vi "AnaBuse_Q1.vi"() -> ()   [LabVIEW 2019]
uses:
  <vilib>/measure/matone.llb/Extract Multiple Tone Information 1 Chan.vi
  <vilib>/measure/NI_MAPro.lvlib
panel:
  out "DHT máximo de  de 10%":bool
  out "DHT":dbl
  in  "stop":bool
  in  "LIGAR":bool
  in  "file path":path=path "C:/lista2.tdms"
  out "SINAL DE TENSAO DA REDE":waveform(dbl)(graph)
  out "multiple tone information":T1(array[cluster]) {"detected phase (deg)" format="%_6g"; "detected amplitude" format="%_6p"; "detected frequency" format="%_6p"}
  # "DHT está dentro das normas?"
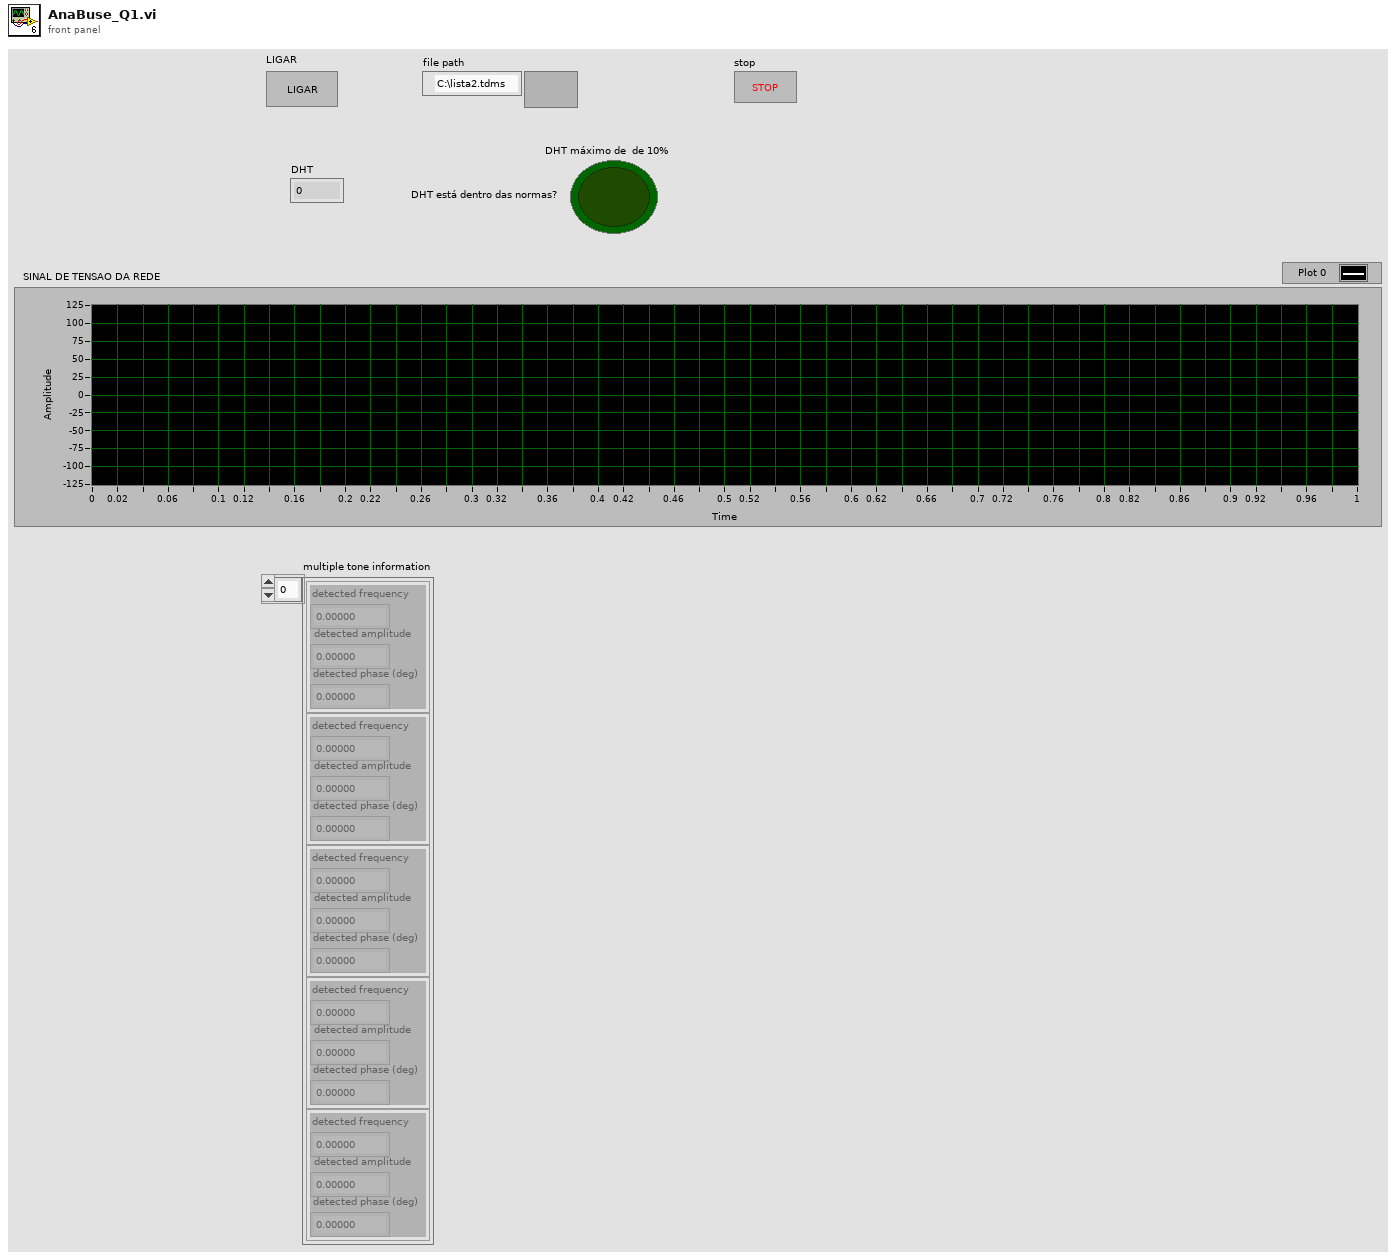
[diagram p1: front panel]
types:
  T1 = cluster{"detected frequency":dbl, "detected amplitude":dbl, "detected phase (deg)":dbl}[]
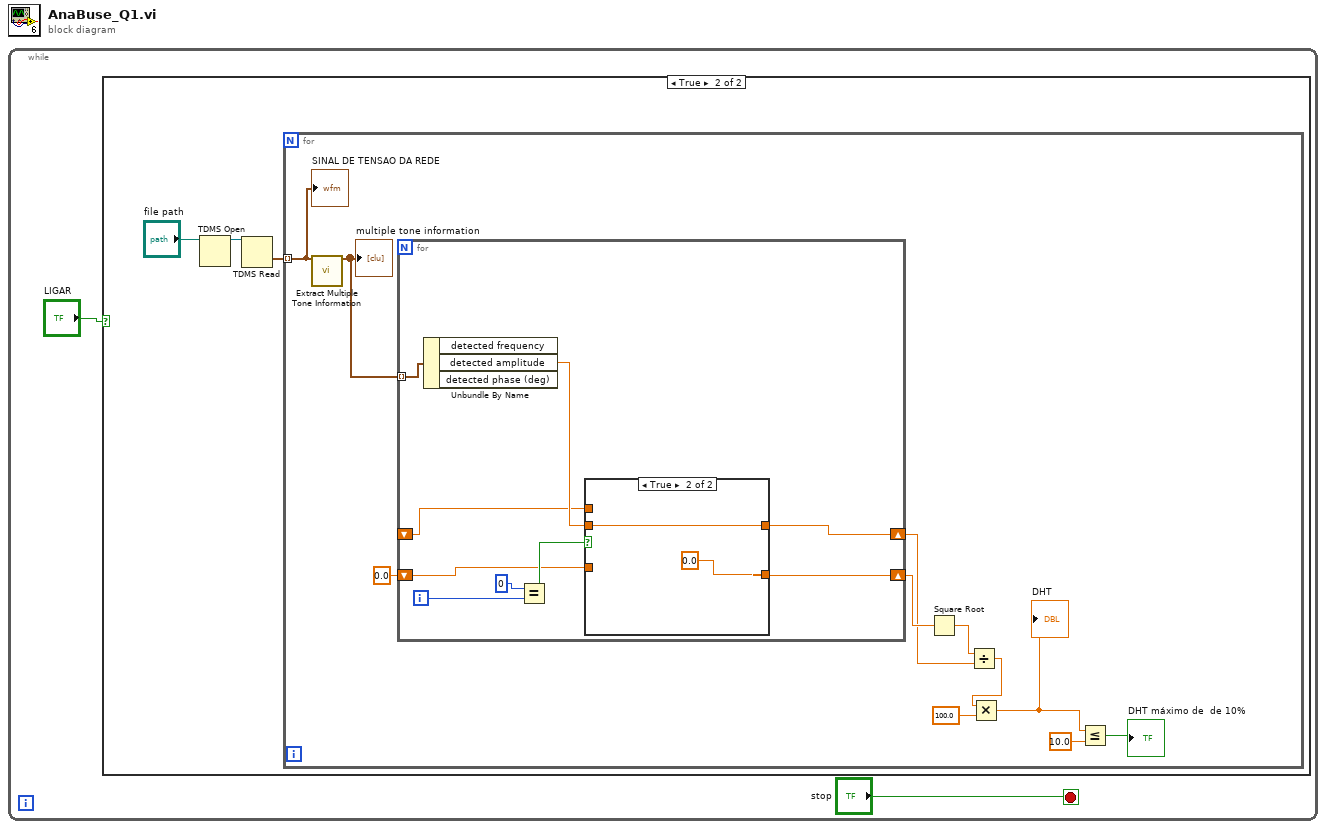
[diagram p0: block diagram]
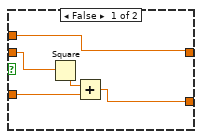
[diagram p3: hidden frame]
diagram:
  n1 = while {
    stop <- "stop" stop-if-true
    n2 = case shown="True" "LIGAR" {
      frame False {
      }
      frame True {
        n3 = TDMS Open(11:"file path") -> (3:w4:refnum<k34>)  [unwired: 6 in, 1 out]
        n4 = TDMS Read(0:w4) -> (10:w3:waveform(dbl)[])  [unwired: 7 in, 5 out]
        n5 = for {
          tunnel: w3 -> [w16] mode=indexing
          n6 = call-poly <vilib>:"Extract Multiple Tone Information.vi"("time signal in"=w16) -> ("multiple tone information"=w15:T1)  [unwired: 12 in, 2 out]
          "multiple tone information" <- w15
          n7 = for {
            tunnel: w15 -> [w25] mode=indexing
            shift-right: [w20] -> w14
            shift-left: 0.0 -> [w19]
            shift-right: [w18] -> w11
            shift-left: _ -> [w17]
            i -> [w22]
            n8 = Unbundle By Name(w25) -> ("detected amplitude"=w24:dbl)  [unwired: 2 out]
            n9 = Equal?(x=0, y=w22) -> (x = y?=w23:bool)
            n10 = case shown="True" w23 {
              tunnel: w24 -> [w30 w32]
              tunnel: [w29 0.0] -> w20
              tunnel: w19 -> [w27 _]
              tunnel: [w26 w32] -> w18
              tunnel: w17 -> [w26 _]
              frame False {
                n11 = Square(x=w30) -> (x^2=w28:dbl)
                n12 = Add(x=w28, y=w27) -> (x+y=w29:dbl)
              }
              frame True {
              }
            }
          }
          n13 = Square Root(x=w14) -> (sqrt(x)=w13:dbl)
          n14 = Divide(x=w13, y=w11) -> (x/y=w10:dbl)
          n15 = Multiply(x=w10, y=100.0) -> (x*y=w6:dbl)
          "DHT" <- w6
          n16 = Less Or Equal?(x=w6, y=10.0) -> (x <= y?=→"DHT máximo de  de 10%":bool)
          "SINAL DE TENSAO DA REDE" <- w16
        }
      }
    }
  }
